vi "DR200-control B_read.vi"(2 "sweep rate (T/min)":dbl, 3 "set field (T)":dbl, 4 "VISA Refnum in":refnum<visa-resource-name>) -> (0 "Field (T)":dbl, 1 "VISA resource name":refnum<visa-resource-name>)   [LabVIEW 2016]
uses:
  IPS120 - SubVIs/IPS-120.lvlib
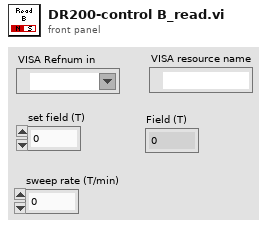
[diagram p1: front panel]
types:
  T1 = cluster{"Field (T)":dbl, "Sweep rate (T/min)":dbl}
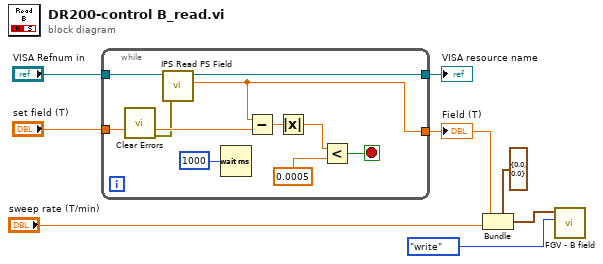
[diagram p0: block diagram]
diagram:
  n1 = while {
    tunnel: "set field (T)" -> [w15]
    tunnel: "VISA Refnum in" -> [w14]
    tunnel: [w13] -> w6
    tunnel: [w10] -> w4
    stop <- w17 stop-if-true
    n2 = call <vilib>:"Clear Errors.vi"() -> ("error out"=w9:errorcluster)  [unwired: 6 in, 1 out]
    n3 = call "IPS Read PS Field.vi"("Error In"=w9, "VISA resource name"=w14) -> ("Field (T)"=w10:dbl, "VISA resource name"=w13:refnum<visa-resource-name>)  [unwired: 3 in, 1 out]
    n4 = Wait (ms)(milliseconds to wait=u32 1000) -> ()  [unwired: 1 out]
    n5 = Subtract(x=w10, y=w15) -> (x-y=w18:dbl)
    n6 = Absolute Value(x=w18) -> (abs(x)=w12:dbl)
    n7 = Less?(x=w12, y=0.0005) -> (x < y?=w17:bool)
  }
  "VISA resource name" <- w6
  "Field (T)" <- w4
  n8 = Bundle(cluster=T1 {"Field (T)"=0.0, "Sweep rate (T/min)"=0.0} ("output cluster"), "Field (T)"=w4, "Sweep rate (T/min)"="sweep rate (T/min)") -> (w2:T1)
  n9 = call "FGV - B field.vi"("Function"=enum16{"write", "read"}."write", "output cluster"=w2) -> ()  [unwired: 4 in, 2 out]
